vi "AB_Log_FileIO.vi"(6 "file":path, 7 "fileAction":T1, 8 "error in (no error)":errorcluster, 10 "data":string, 11 "newSection":string) -> (0 "error out":errorcluster)   [LabVIEW 2020]
uses:
  <vilib>/AppBuilder/logging/AB_Log_File_Action.ctl
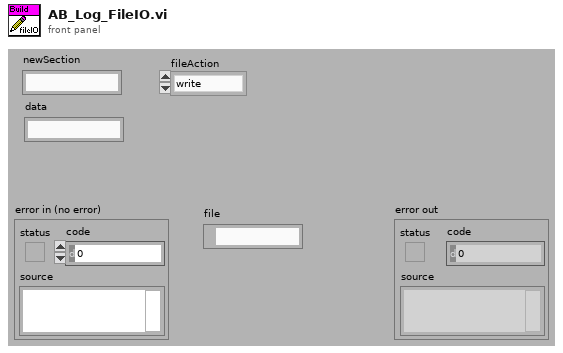
[diagram p1: front panel]
types:
  T1 = typedef "AB_Log_File_Action.ctl" = enum16{"write", "open", "close"}
  T2 = enum16{"open", "open or create", "create or replace", "create", "open (read only)"}
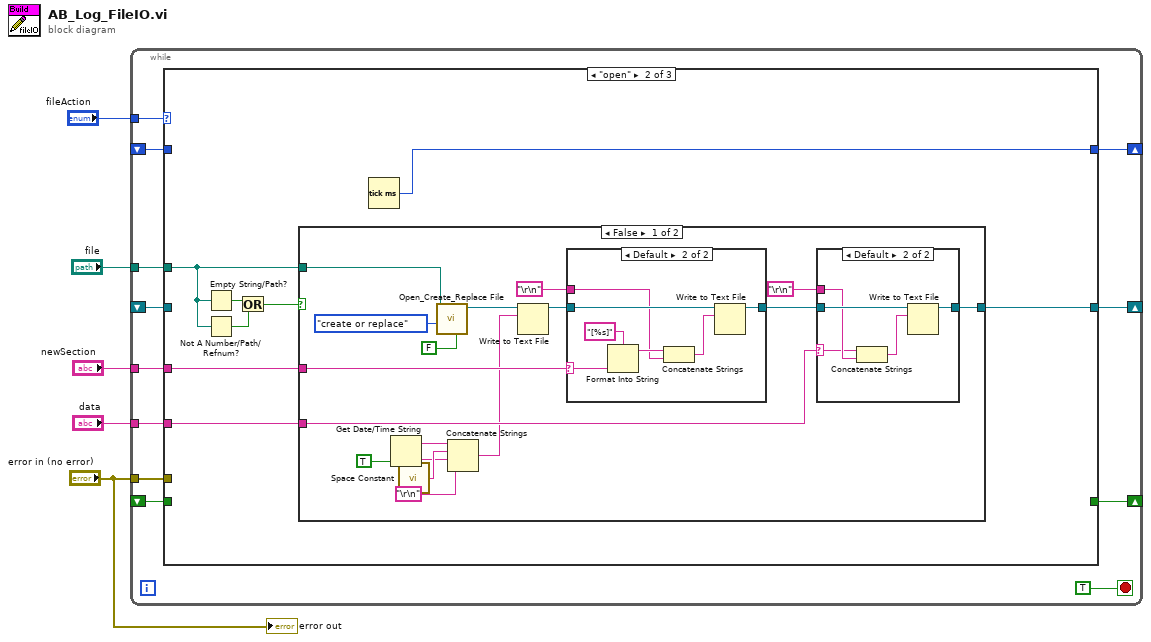
[diagram p0: block diagram]
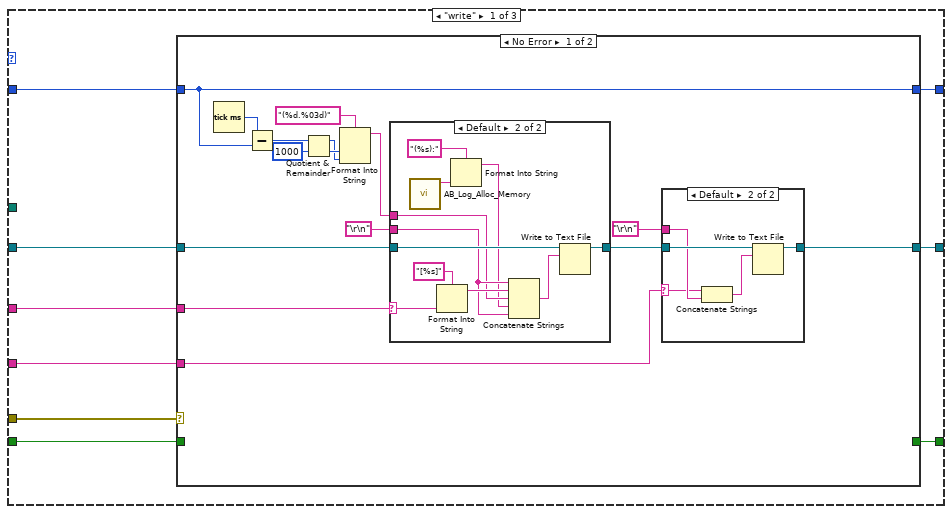
[diagram p2: hidden frame]
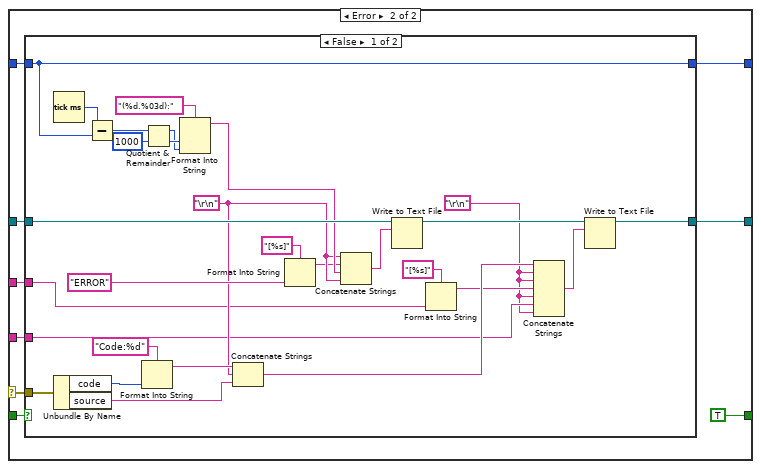
[diagram p5: hidden frame]
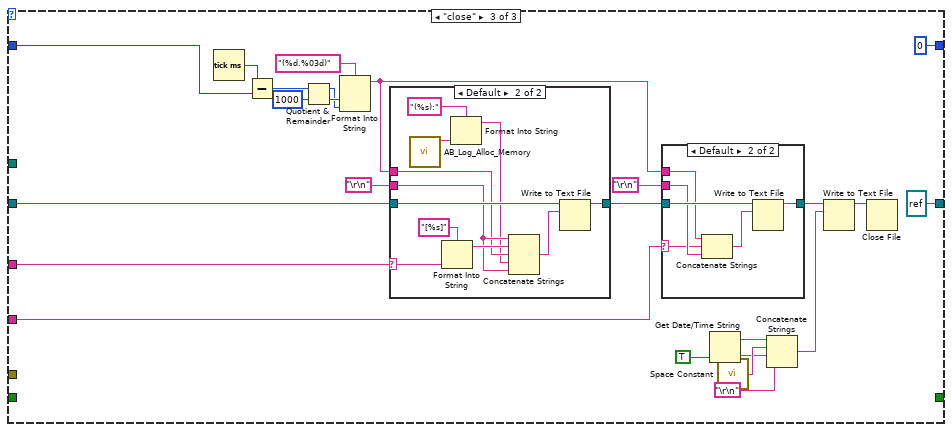
[diagram p10: hidden frame]
diagram:
  n1 = while {
    tunnel: "fileAction" -> [w16]
    shift-right: [w15] -> _
    shift-left: _ -> [w12]
    tunnel: "file" -> [w14]
    shift-right: [w13] -> _
    shift-left: _ -> [w9]
    tunnel: "newSection" -> [w11]
    tunnel: "data" -> [w10]
    tunnel: "error in (no error)" -> [w8]
    shift-right: [w7] -> _
    shift-left: _ -> [w6]
    stop <- TRUE stop-if-true
    n2 = case shown="\"open\"" w16 {
      tunnel: [w18 w103 u32 0 ("millisecond timer value")] -> w15
      tunnel: w14 -> [_ w102 _]
      tunnel: [w26 w106 refnum<file> refnum ("refnum out")] -> w13
      tunnel: w12 -> [w22 _ w158]
      tunnel: w11 -> [w23 w104 w159]
      tunnel: w10 -> [w25 w105 w161]
      tunnel: w9 -> [w24 _ w160]
      tunnel: w8 -> [w21 _ _]
      tunnel: [w20 _ _] -> w7
      tunnel: w6 -> [w19 _ _]
      frame "write" {
        n3 = case shown="No Error" w21 {
          selector: w21 -> [_ w61]
          tunnel: [w28 w64] -> w26
          tunnel: w25 -> [w32 w65]
          tunnel: w24 -> [w35 w68]
          tunnel: w23 -> [w34 w67]
          tunnel: w22 -> [w27 w66]
          tunnel: [_ TRUE] -> w20
          tunnel: w19 -> [_ w62]
          tunnel: [w27 w60] -> w18
          frame No Error {
            n4 = Tick Count (ms)() -> (millisecond timer value=w41:u32)
            n5 = Subtract(x=w41, y=w27) -> (x-y=w39:u32)
            n6 = Quotient & Remainder(x=w39, y=u32 1000) -> (x-y*floor(x/y)=w36:u32, floor(x/y)=w37:u32)
            n7 = Format Into String(format string="(%d.%03d)", w37, w36) -> (resulting string=w31:string)  [unwired: 2 in, 1 out]
            n8 = case shown="Default" w34 {
              selector: w34 -> [_ w55]
              tunnel: w35 -> [w48 w59]
              tunnel: [w48 w58] -> w29
              tunnel: "\r\n" -> [_ w53]
              tunnel: w31 -> [_ w52]
              frame "" {
              }
              frame Default {
                n9 = call <vilib>:"AB_Log_Alloc_Memory.vi"() -> ("memory blocks"=w51:string)  [unwired: 10 in, 1 out]
                n10 = Format Into String(format string="[%s]", w55) -> (resulting string=w54:string)  [unwired: 2 in, 1 out]
                n11 = Format Into String(format string="(%s):", w51) -> (resulting string=w49:string)  [unwired: 2 in, 1 out]
                n12 = Concatenate Strings(w53, w54, w52, w49, w53) -> (w57:string)
                n13 = Write to Text File(file (use dialog)=w59, text=w57) -> (refnum out=w58:refnum<file>)  [unwired: 2 in, 2 out]
              }
            }
            n14 = case shown="Default" w32 {
              selector: w32 -> [_ w43]
              tunnel: w29 -> [w42 w47]
              tunnel: [w42 w46] -> w28
              tunnel: "\r\n" -> [_ w44]
              frame "" {
              }
              frame Default {
                n15 = Concatenate Strings(w43, w44) -> (w45:string)
                n16 = Write to Text File(file (use dialog)=w47, text=w45) -> (refnum out=w46:refnum<file>)  [unwired: 2 in, 2 out]
              }
            }
          }
          frame Error {
            n17 = case shown="False" w62 {
              tunnel: w68 -> [w90 w98]
              tunnel: w67 -> [w71 _]
              tunnel: w66 -> [w78 w97]
              tunnel: w65 -> [w73 _]
              tunnel: [w87 w98] -> w64
              tunnel: w61 -> [w86 _]
              tunnel: [w78 w97] -> w60
              frame False {
                w69 = "\r\n"
                w81 = "\r\n"
                n18 = Tick Count (ms)() -> (millisecond timer value=w96:u32)
                n19 = Unbundle By Name(w86) -> ("code"=w83:i32, "source"=w80:string)
                n20 = Subtract(x=w96, y=w78) -> (x-y=w94:u32)
                n21 = Format Into String(format string="Code:%d", w83) -> (resulting string=w82:string)  [unwired: 2 in, 1 out]
                n22 = Quotient & Remainder(x=w94, y=u32 1000) -> (x-y*floor(x/y)=w91:u32, floor(x/y)=w92:u32)
                n23 = Format Into String(format string="(%d.%03d):", w92, w91) -> (resulting string=w89:string)  [unwired: 2 in, 1 out]
                n24 = Concatenate Strings(w82, w81, w80) -> (w79:string)
                n25 = Format Into String(format string="[%s]", "ERROR" ("format string")) -> (resulting string=w74:string)  [unwired: 2 in, 1 out]
                n26 = Concatenate Strings(w81, w74, w89, w81) -> (w76:string)
                n27 = Write to Text File(file (use dialog)=w90, text=w76) -> (refnum out=w88:refnum<file>)  [unwired: 2 in, 2 out]
                n28 = Format Into String(format string="[%s]", w71) -> (resulting string=w70:string)  [unwired: 2 in, 1 out]
                n29 = Concatenate Strings(w79, w69, w69, w70, w69, w73, w69) -> (w77:string)
                n30 = Write to Text File(file (use dialog)=w88, text=w77) -> (refnum out=w87:refnum<file>)  [unwired: 2 in, 2 out]
              }
              frame True {
              }
            }
          }
        }
      }
      frame "open" {
        n31 = Empty String/Path?(string/path=w102) -> (empty?=w101:bool)
        n32 = Not A Number/Path/Refnum?(number/path/refnum=w102) -> (NaN/Path/Refnum?=w100:bool)
        n33 = Or(x=w101, y=w100) -> (x .or. y?=w99:bool)
        n34 = case shown="False" w99 {
          tunnel: [w123 _] -> w106
          tunnel: w105 -> [w122 _]
          tunnel: w104 -> [w121 _]
          tunnel: w102 -> [w107 _]
          frame False {
            n35 = Get Date/Time String(want seconds? (F)=TRUE) -> (date string=w112:string, time string=w110:string)  [unwired: 2 in]
            n36 = call <vilib>:"Space Constant.vi"() -> ("String"=w111:string)
            n37 = call <vilib>:"Open_Create_Replace File.vi"("advisory dialog? (display:T)"=FALSE, "function (open:0)"=T2."create or replace", "file path"=w107) -> ("refnum"=w115:refnum<file>)  [unwired: 5 in, 3 out]
            n38 = Concatenate Strings(w112, w111, w110, "\r\n") -> (w108:string)
            n39 = Write to Text File(file (use dialog)=w115, text=w108) -> (refnum out=w114:refnum<file>)  [unwired: 2 in, 2 out]
            n40 = case shown="Default" w121 {
              selector: w121 -> [_ w133]
              tunnel: w114 -> [w130 w137]
              tunnel: [w130 w136] -> w118
              tunnel: "\r\n" -> [_ w131]
              frame "" {
              }
              frame Default {
                n41 = Format Into String(format string="[%s]", w133) -> (resulting string=w132:string)  [unwired: 2 in, 1 out]
                n42 = Concatenate Strings(w132, w131) -> (w135:string)
                n43 = Write to Text File(file (use dialog)=w137, text=w135) -> (refnum out=w136:refnum<file>)  [unwired: 2 in, 2 out]
              }
            }
            n44 = case shown="Default" w122 {
              selector: w122 -> [_ w125]
              tunnel: w118 -> [w124 w129]
              tunnel: [w124 w128] -> w123
              tunnel: "\r\n" -> [_ w126]
              frame "" {
              }
              frame Default {
                n45 = Concatenate Strings(w125, w126) -> (w127:string)
                n46 = Write to Text File(file (use dialog)=w129, text=w127) -> (refnum out=w128:refnum<file>)  [unwired: 2 in, 2 out]
              }
            }
          }
          frame True {
          }
        }
        n47 = Tick Count (ms)() -> (millisecond timer value=w103:u32)
      }
      frame "close" {
        n48 = Tick Count (ms)() -> (millisecond timer value=w157:u32)
        n49 = Subtract(x=w157, y=w158) -> (x-y=w155:u32)
        n50 = Quotient & Remainder(x=w155, y=u32 1000) -> (x-y*floor(x/y)=w152:u32, floor(x/y)=w153:u32)
        n51 = Format Into String(format string="(%d.%03d)", w153, w152) -> (resulting string=w150:string)  [unwired: 2 in, 1 out]
        n52 = case shown="Default" w159 {
          selector: w159 -> [_ w176]
          tunnel: w160 -> [w169 w180]
          tunnel: [w169 w179] -> w148
          tunnel: "\r\n" -> [_ w174]
          tunnel: w150 -> [_ w173]
          frame "" {
          }
          frame Default {
            n53 = call <vilib>:"AB_Log_Alloc_Memory.vi"() -> ("memory blocks"=w171:string)  [unwired: 10 in, 1 out]
            n54 = Format Into String(format string="[%s]", w176) -> (resulting string=w175:string)  [unwired: 2 in, 1 out]
            n55 = Format Into String(format string="(%s):", w171) -> (resulting string=w170:string)  [unwired: 2 in, 1 out]
            n56 = Concatenate Strings(w174, w175, w173, w170, w174) -> (w178:string)
            n57 = Write to Text File(file (use dialog)=w180, text=w178) -> (refnum out=w179:refnum<file>)  [unwired: 2 in, 2 out]
          }
        }
        n58 = case shown="Default" w161 {
          selector: w161 -> [_ w164]
          tunnel: w148 -> [w162 w168]
          tunnel: [w162 w167] -> w142
          tunnel: "\r\n" -> [_ w165]
          tunnel: w150 -> [_ w163]
          frame "" {
          }
          frame Default {
            n59 = Concatenate Strings(w163, w164, w165) -> (w166:string)
            n60 = Write to Text File(file (use dialog)=w168, text=w166) -> (refnum out=w167:refnum<file>)  [unwired: 2 in, 2 out]
          }
        }
        n61 = Get Date/Time String(want seconds? (F)=TRUE) -> (date string=w146:string, time string=w144:string)  [unwired: 2 in]
        n62 = call <vilib>:"Space Constant.vi"() -> ("String"=w145:string)
        n63 = Concatenate Strings(w146, w145, w144, "\r\n") -> (w140:string)
        n64 = Write to Text File(file (use dialog)=w142, text=w140) -> (refnum out=w141:refnum<file>)  [unwired: 2 in, 2 out]
        n65 = Close File(refnum=w141) -> ()  [unwired: 1 in, 2 out]
      }
    }
  }
  "error out" <- "error in (no error)"
